vi "_TreeItem.Property.Set.Dictionary.Write.vi"(8 "error in (no error)":errorcluster, 11 "Dictionary":T1) -> (0 "error out":errorcluster, 3 "DictionaryProperty":refnum<k24>)   [LabVIEW 2016, in "Advanced System Definition.lvlib"]
uses:
  SysDef API/Advanced System Definition.lvlib
  NationalInstruments.VeriStand.SystemStorage
  _Types/Property.Dictionary.ctl
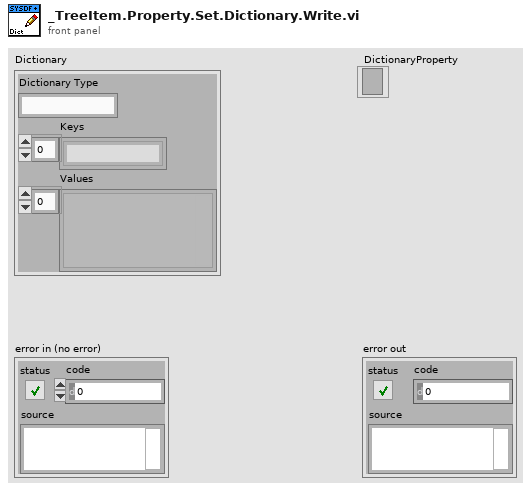
[diagram p1: front panel]
types:
  T1 = typedef "Advanced System Definition.lvlib/Property.Dictionary.ctl" = cluster{"Dictionary Type":string, "Keys":string[], "Values":variant[]}
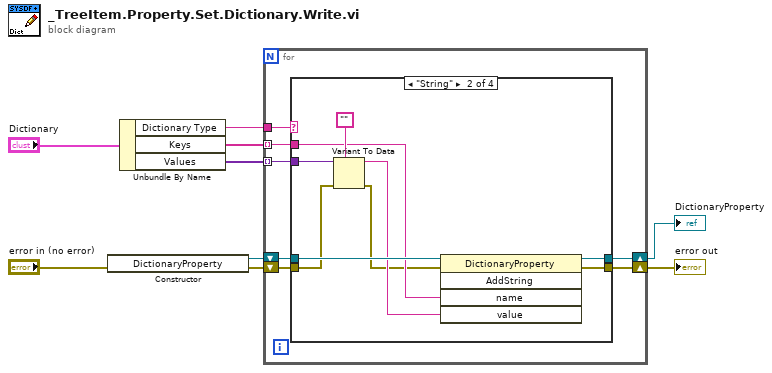
[diagram p0: block diagram]
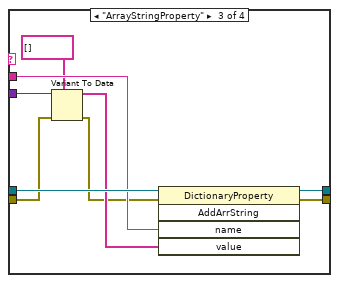
[diagram p3: hidden frame]
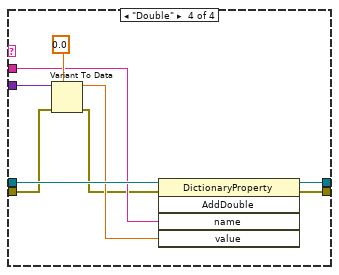
[diagram p4: hidden frame]
diagram:
  n1 = constructor class="DictionaryProperty"(error in="error in (no error)") -> (reference out=w9:refnum<k24>, error out=w4:errorcluster)  [unwired: 2 in, 1 out]
  n2 = Unbundle By Name("Dictionary") -> ("Dictionary Type"=w8:string, "Keys"=w5:string[], "Values"=w6:variant[])
  n3 = for {
    shift-right: [w15] -> w1
    shift-left: w9 -> [w16]
    tunnel: w8 -> [w14]
    tunnel: w6 -> [w13] mode=indexing
    tunnel: w5 -> [w12] mode=indexing
    shift-right: [w10] -> w2
    shift-left: w4 -> [w11]
    n4 = case shown="\"String\"" w14 {
      tunnel: w16 -> [w18 w26 w36 w44]
      tunnel: [w18 w24 w34 w42] -> w15
      tunnel: w12 -> [_ w22 w32 w40]
      tunnel: w13 -> [_ w23 w33 w41]
      tunnel: w11 -> [w17 w21 w31 w39]
      tunnel: [w17 w19 w29 w37] -> w10
      frame Default {
      }
      frame "String" {
        n5 = Variant To Data(error in=w21, type="", Variant=w23) -> (data=w25:string, error out=w20:errorcluster)
        n6 = invoke class="DictionaryProperty" method="AddString"(reference=w26, error in=w20, "name"=w22, "value"=w25) -> (reference out=w24:refnum<k24>, error out=w19:errorcluster)  [unwired: 1 in, 3 out]
      }
      frame "ArrayStringProperty" {
        n7 = Variant To Data(error in=w31, type=string[] [], Variant=w33) -> (data=w35:string[], error out=w30:errorcluster)
        n8 = invoke class="DictionaryProperty" method="AddArrString"(reference=w36, error in=w30, "name"=w32, "value"=w35) -> (reference out=w34:refnum<k24>, error out=w29:errorcluster)  [unwired: 1 in, 3 out]
      }
      frame "Double" {
        n9 = Variant To Data(error in=w39, type=0.0, Variant=w41) -> (data=w43:dbl, error out=w38:errorcluster)
        n10 = invoke class="DictionaryProperty" method="AddDouble"(reference=w44, error in=w38, "name"=w40, "value"=w43) -> (reference out=w42:refnum<k24>, error out=w37:errorcluster)  [unwired: 1 in, 3 out]
      }
    }
  }
  "error out" <- w2
  "DictionaryProperty" <- w1
